vi "Verify Adaptive Drain time.vi"(0 "GEA2 Reference In":refnum<k24>, 5 "ECT Data In":T1, 11 "Error In":errorcluster) -> (3 "Expected SSD":string, 4 "GEA2 Reference Out":refnum<k24>, 6 "Actual ECT After Drain (sec)":u16, 8 "Expected ECT After Drain(sec)":u16, 10 "ECT After Drain Pass/Fail":bool, 14 "Report Text":string, 15 "Error Out":errorcluster)   [LabVIEW 2016, in "TLMB.lvlib"]
doc: "This vi can be used to read ERD every 1 sec for user selected repeat counts."
uses:
  Projects/TLMB.lvlib
  Q:/Common/DLLs/GEA3/GeaCommunication.dll
  Common/DLLs/GEA3/GeaCommunication.dll
  Controls/ECT.ctl
  Common/LabVIEW GEA2 Toolkit/LabVIEW_GEA2_Toolkit.lvlibp/type defs/Source_Destination.ctl
  Common/LabVIEW GEA2 Toolkit/LabVIEW_GEA2_Toolkit.lvlibp/type defs/ERD Read Data In.ctl
  Common/LabVIEW GEA2 Toolkit/LabVIEW_GEA2_Toolkit.lvlibp/type defs/Data Type.ctl
  Common/LabVIEW GEA2 Toolkit/LabVIEW_GEA2_Toolkit.lvlibp
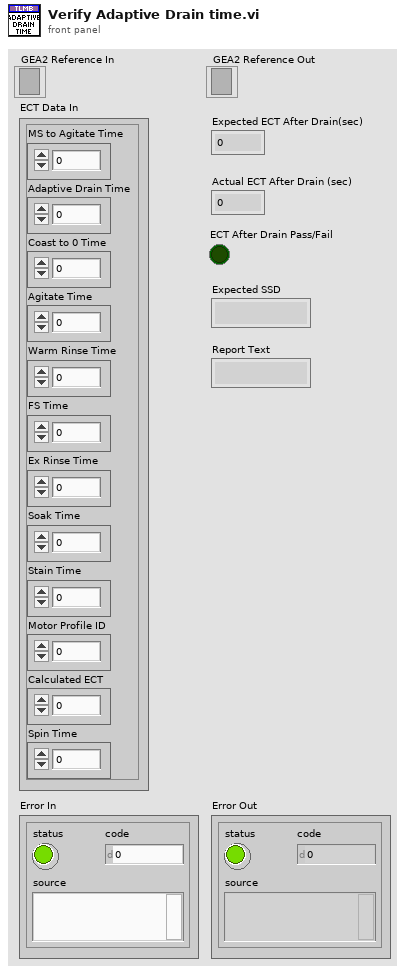
[diagram p1: front panel]
types:
  T1 = typedef "TLMB.lvlib/ECT.ctl" = cluster{"MS to Agitate Time":u16, "Adaptive Drain Time":u16, "Coast to 0 Time":u16, "Agitate Time":u16, "Warm Rinse Time":u16, "FS Time":u16, "Ex Rinse Time":u16, "Soak Time":u16, "Stain Time":u16, "Motor Profile ID":u16, "Calculated ECT":u16, "Spin Time":u16}
  T2 = typedef "LabVIEW_GEA2_Toolkit.lvlibp/Source_Destination.ctl" = cluster{"Source":u8, "Destination":u8}
  T3 = typedef "LabVIEW_GEA2_Toolkit.lvlibp/ERD Read Data In.ctl" = cluster{"ERD Number":u16, "Data Type":T4}
  T4 = typedef "LabVIEW_GEA2_Toolkit.lvlibp/Data Type.ctl" = enum16{"string", "boolean", "uint8_t", "uint16_t", "uint32_t", "uint64_t", "int8_t", "int16_t", "int32_t", "int64_t"}
  T5 = enum16{"EQ (==)", "NE (!=)", "GT (>)", "LT (<)", "GE (>=)", "LE (<=)", "GTLT(> <)", "GELE (>= <=)", "GELT (>= <)", "GTLE (> <=)", "LTGT (< >)", "LEGE (<= >=)", "LEGT (<= >)", "LTGE (< >=)", "No Comparison"}
  T6 = typedef "LabVIEW_GEA2_Toolkit.lvlibp/ERD Read Data Out.ctl" = cluster{"ERD Number":u16, "Data":string}
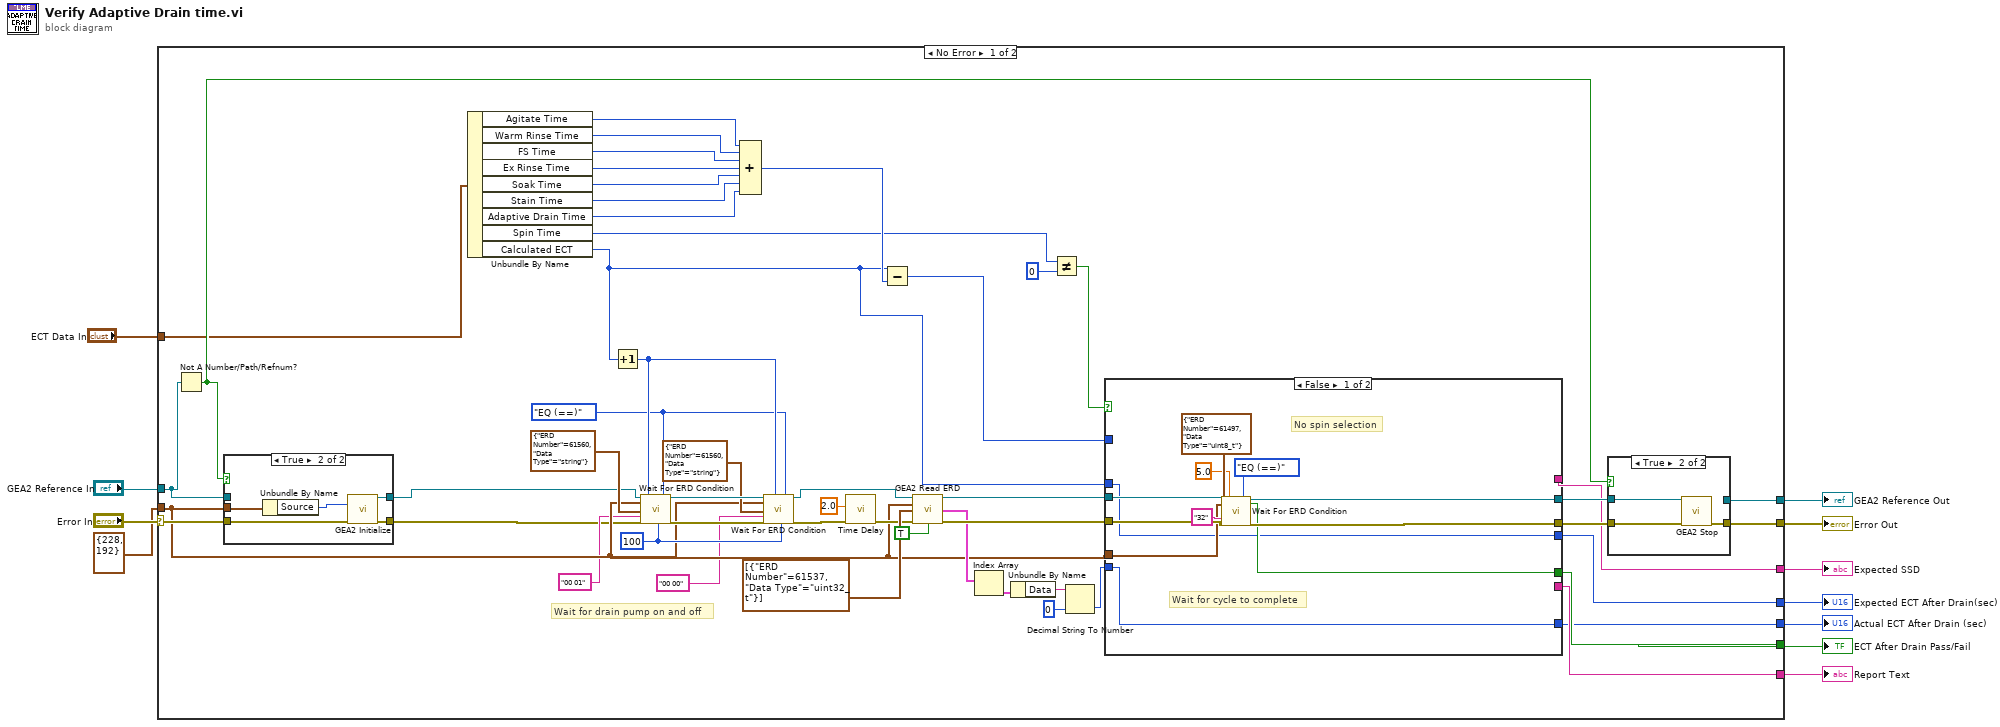
[diagram p0: block diagram]
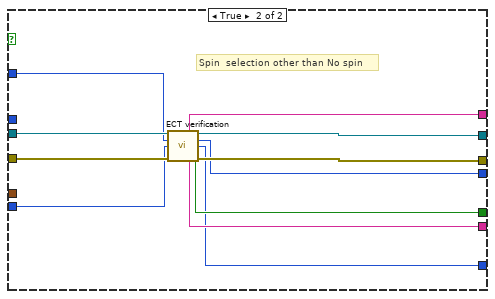
[diagram p2: hidden frame]
diagram:
  n1 = case shown="No Error" "Error In" {
    selector: "Error In" -> [w61 w98]
    tunnel: T2 {"Source"=228, "Destination"=192} ("GEA Inputs") -> [w23 _]
    tunnel: "GEA2 Reference In" -> [w62 w99]
    tunnel: [w58 w99] -> w9
    tunnel: [w60 w98] -> w8
    tunnel: "ECT Data In" -> [w12 _]
    tunnel: [w34 _] -> w6
    tunnel: [w33 _] -> w5
    tunnel: [w32 _] -> w4
    tunnel: [w31 _] -> w3
    tunnel: [w19 _] -> w1
    frame No Error {
      w16 = T5."EQ (==)" ("Comparison")
      w50 = u32 100 ("Loop Rate (ms)")
      # "Wait for drain pump on and off"
      n2 = Not A Number/Path/Refnum?(number/path/refnum=w62) -> (NaN/Path/Refnum?=w59:bool)
      n3 = case shown="True" w59 {
        tunnel: w61 -> [w92 w97]
        tunnel: [w92 w96] -> w13
        tunnel: [w91 w95] -> w24
        tunnel: w23 -> [_ w93]
        tunnel: w62 -> [w91 _]
        frame False {
        }
        frame True {
          n4 = Unbundle By Name(w93) -> ("Source"=w94:u8)
          n5 = call "GEA2 Initialize.vi"("Source Address"=w94, "error in"=w97) -> ("GEA2 Reference Out"=w95:refnum<k24>, "error out"=w96:errorcluster)  [unwired: 11 in, 1 out]
        }
      }
      n6 = Unbundle By Name(w12) -> ("Agitate Time"=w43:u16, "Warm Rinse Time"=w42:u16, "FS Time"=w41:u16, "Ex Rinse Time"=w40:u16, "Soak Time"=w39:u16, "Stain Time"=w38:u16, "Adaptive Drain Time"=w35:u16, "Spin Time"=w15:u16, "Calculated ECT"=w14:u16)
      n7 = Increment(x=w14) -> (x+1=w22:u16)
      n8 = call "Wait For ERD Condition.vi"("GEA2 Reference In"=w24, "GEA Inputs"=w23, "ERD Read Data"=T3 {"ERD Number"=61560, "Data Type"=enum."string"}, "Expected Low"="00 01" ("string"), "Error In"=w13, "Timeout (s)"=w22, "Loop Rate (ms)"=w50, "Comparison"=w16) -> ("GEA2 Reference Out"=w53:refnum<k24>, "Error Out"=w52:errorcluster)  [unwired: 7 in, 3 out]
      n9 = Compound Arithmetic op=ADD(w43, w42, w41, w40, w39, w38, w35) -> (w37:u16)
      n10 = call "Wait For ERD Condition.vi"("GEA2 Reference In"=w53, "GEA Inputs"=w23, "ERD Read Data"=T3 {"ERD Number"=61560, "Data Type"=enum."string"}, "Expected Low"="00 00" ("string"), "Error In"=w52, "Timeout (s)"=w22, "Loop Rate (ms)"=w50, "Comparison"=w16) -> ("GEA2 Reference Out"=w51:refnum<k24>, "Error Out"=w47:errorcluster)  [unwired: 7 in, 3 out]
      n11 = call "Time Delay"("error in (no error)"=w47, "Delay Time (s)"=2.0) -> ("error out"=w46:errorcluster)  [unwired: 9 in]
      n12 = Subtract(x=w14, y=w37) -> (x-y=w36:u16)
      n13 = call "GEA2 Read ERD.vi"("GEA2 Reference In"=w51, "GEA Inputs"=w23, "Read ERD List"=T3[] [{"ERD Number"=61537, "Data Type"=enum."uint32_t"}], "Error In"=w46, "Verify ERD Response?"=TRUE) -> ("GEA2 Reference Out"=w30:refnum<k24>, "ERD Data Out"=w28:T6[], "Error Out"=w29:errorcluster)  [unwired: 7 in, 1 out]
      n14 = Index Array(array=w28) -> (element=w27:T6)  [unwired: 1 in]
      n15 = Unbundle By Name(w27) -> ("Data"=w26:string)
      n16 = Not Equal?(x=w15, y=u16 0) -> (x != y?=w44:bool)
      n17 = Decimal String To Number(string=w26, default (0L)=u16 0 ("Actual ECT After Drain (sec)")) -> (number=w25:u16)  [unwired: 1 in, 1 out]
      n18 = case shown="False" w44 {
        tunnel: [w67 w85] -> w56
        tunnel: [w66 w84] -> w55
        tunnel: w36 -> [_ w77]
        tunnel: [_ w83] -> w31
        tunnel: [w65 w82] -> w32
        tunnel: [w63 w81] -> w33
        tunnel: [_ w80] -> w34
        tunnel: w23 -> [w68 _]
        tunnel: w30 -> [w74 w79]
        tunnel: w29 -> [w73 w78]
        tunnel: w14 -> [w63 _]
        tunnel: w25 -> [w64 w76]
        tunnel: [w64 w75] -> w19
        frame False {
          # "Wait for cycle to complete"
          # "No spin selection"
          n19 = call "Wait For ERD Condition.vi"("GEA2 Reference In"=w74, "GEA Inputs"=w68, "ERD Read Data"=T3 {"ERD Number"=61497, "Data Type"=enum."uint8_t"}, "Expected Low"="32", "Error In"=w73, "Timeout (s)"=5.0, "Comparison"=T5."EQ (==)") -> ("GEA2 Reference Out"=w67:refnum<k24>, "Pass/Fail?"=w65:bool, "Error Out"=w66:errorcluster)  [unwired: 8 in, 2 out]
        }
        frame True {
          # "Spin  selection other than No spin"
          n20 = call "ECT verification.vi"(".NET Refnum in"=w79, "Cal ECT (sec)"=w77, "Time remaining (sec)"=w76, "error in"=w78) -> ("Expected SSD"=w80:string, ".NET Refnum out"=w85:refnum<k24>, "Expected ECT (sec)"=w81:u16, "Actual ECT (sec)"=w75:u16, "ECT Pass/Fail"=w82:bool, "Report Text"=w83:string, "error out"=w84:errorcluster)  [unwired: 5 in]
        }
      }
      n21 = case shown="True" w59 {
        tunnel: [w87 w90] -> w60
        tunnel: w56 -> [w86 w89]
        tunnel: w55 -> [w87 w88]
        tunnel: [w86 _] -> w58
        frame False {
        }
        frame True {
          n22 = call "GEA2 Stop.vi"("GEA2 Reference In"=w89, "Error In"=w88) -> ("Error Out"=w90:errorcluster)  [unwired: 13 in]
        }
      }
    }
    frame Error {
    }
  }
  "GEA2 Reference Out" <- w9
  "Error Out" <- w8
  "Expected SSD" <- w6
  "Expected ECT After Drain(sec)" <- w5
  "Actual ECT After Drain (sec)" <- w1
  "ECT After Drain Pass/Fail" <- w4
  "Report Text" <- w3
